vi "Get Columns.vi"(8 "error in (no error)":errorcluster, 10 "Table Path":string, 11 "Data.PG":refnum<class "LV-Data.PGSQL.lvclass">) -> (0 "error out":errorcluster, 1 "Column Paths":string[](array[string]), 2 "Column Names":string[](array[string]), 3 "Data.PG out":refnum<class "LV-Data.PGSQL.lvclass">, 4 "Column Units":string[](array[string]))   [LabVIEW 2019, in "LV-Data.PGSQL.lvclass"]
uses:
  LV-Data.PGSQL.lvclass
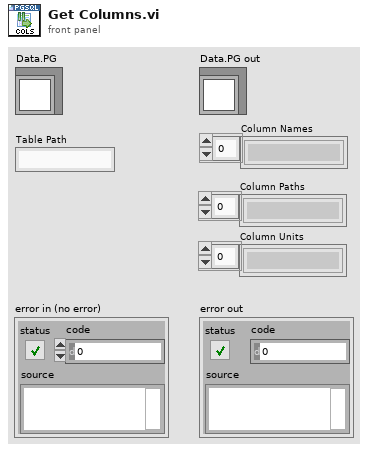
[diagram p1: front panel]
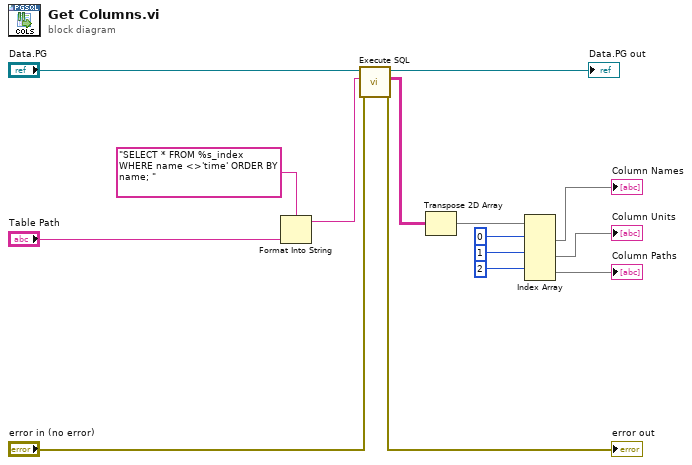
[diagram p0: block diagram]
diagram:
  n1 = Format Into String(format string="SELECT * FROM %s_index WHERE name <>'time' ORDER BY name; ", "Table Path") -> (resulting string=w8:string)  [unwired: 2 in, 1 out]
  n2 = call "Execute SQL.vi"("error in"="error in (no error)", "SQL"=w8, "LV-Data.PGSQL"="Data.PG") -> ("error out"=→"error out":errorcluster, "Result"=w2:string[][], "LV-Data.PGSQL out"=→"Data.PG out":refnum<class "LV-Data.PGSQL.lvclass">)  [unwired: 6 in]
  n3 = Transpose 2D Array(2D array=w2) -> (transposed array=w9:string[][])
  n4 = Index Array(array=w9, index (row) #1=0 ("index (row)"), index (row) #2=1 ("index (row)"), index (row) #3=2 ("index (row)")) -> (element #1=→"Column Names":string[], element #2=→"Column Units":string[], element #3=→"Column Paths":string[])  [unwired: 3 in]
